vi "Refnum Initialize.vi"(8 "error in (no error)":errorcluster, 11 "QTab Class in":refnum<class "QTab Class.lvclass">) -> (0 "error out":errorcluster, 3 "QTab Class out":refnum<class "QTab Class.lvclass">)   [LabVIEW 2020, in "QTab.lvlib" / "QTab Class.lvclass"]
uses:
  QTab Class.lvclass
  Command Data.ctl
  Command.ctl
  Pag Attribute.ctl
  Close Event Data.ctl
  QTab Class.lvclass/QTab Class.ctl
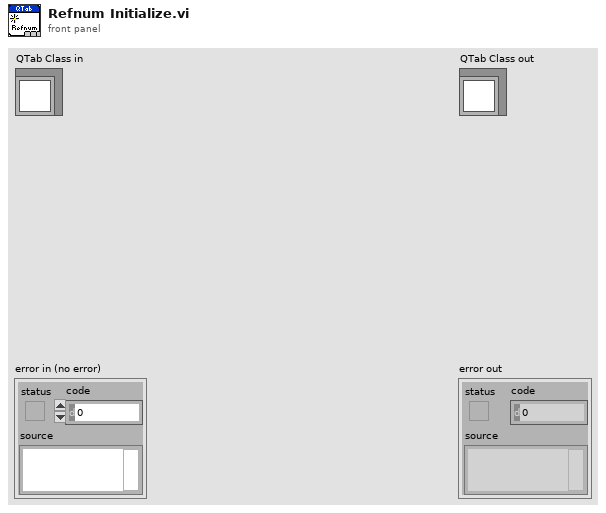
[diagram p1: front panel]
types:
  T1 = typedef "QTab.lvlib/QTab Class.lvclass/Close Event Data.ctl" = cluster{"VI Refnum":refnum<vi>, "Page Name":string, "Confirm Notifier":refnum<notifier>}
  T2 = typedef "QTab.lvlib/QTab Class.lvclass/Pag Attribute.ctl" = cluster{"VI Refnum":refnum<vi>, "Page Name":string, "Closeable":bool, "Draggable":bool, "Pop-Out":bool}
  T3 = typedef "QTab.lvlib/QTab Class.lvclass/Command Data.ctl" = cluster{"Command":T4, "Data":variant}
  T4 = typedef "QTab.lvlib/QTab Class.lvclass/Command.ctl" = enum16{"Startup", "Add Page", "Close All Page", "Set Page Attribute", "Pop-out", "Merage", "Insert", "Stop"}
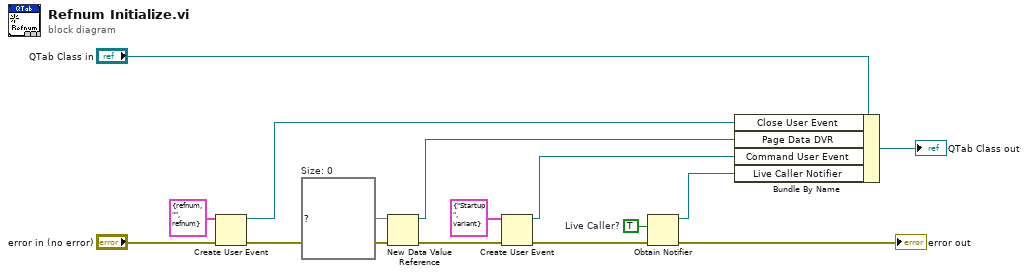
[diagram p0: block diagram]
diagram:
  w7 = map{string, T2} {}  # Size: 0
  w12 = TRUE  # Live Caller?
  n1 = Create User Event(user event datatype=T1 {"VI Refnum"=refnum, "Page Name"="", "Confirm Notifier"=refnum} ("Close Event Data"), error in="error in (no error)") -> (user event=w1:refnum<user-event>, error out=w2:errorcluster)
  n2 = New Data Value Reference(data value=w7, error in=w2) -> (data value reference=w5:refnum<data-value>, error out=w6:errorcluster)
  n3 = Create User Event(user event datatype=T3 {"Command"=enum."Startup", "Data"=variant} ("Command Data"), error in=w6) -> (user event=w10:refnum<user-event>, error out=w11:errorcluster)
  n4 = Obtain Notifier(notification data type=w12, error in (no error)=w11) -> (notifier out=w9:refnum<notifier>, error out=→"error out":errorcluster)  [unwired: 2 in, 1 out]
  n5 = Bundle By Name(cluster="QTab Class in", "Close User Event"=w1, "Page Data DVR"=w5, "Command User Event"=w10, "Live Caller Notifier"=w9) -> (→"QTab Class out":refnum<class "QTab Class.lvclass">)
